vi "lineStartEndInfo.vi"(9 "current location":T1, 10 "line status":cluster{"line start":bool, "line end":bool}, 11 "scan info":T2) -> (3 "scan info out":T2)   [LabVIEW 2010]
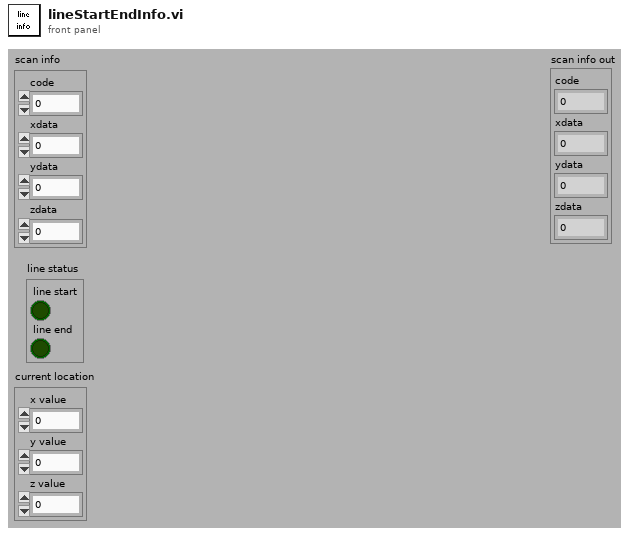
[diagram p1: front panel]
types:
  T1 = cluster{"x value":i16, "y value":i16, "z value":i16}
  T2 = cluster{"code":i32, "xdata":i32, "ydata":i32, "zdata":i32}
  T3 = enum16{"NONE", "VOLUME_START", "LINE_START", "LINE_END", "VOLUME_END"}
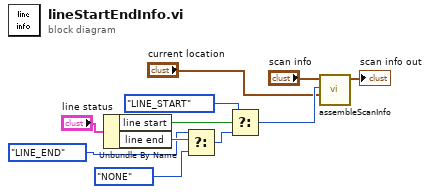
[diagram p0: block diagram]
diagram:
  n1 = Unbundle By Name("line status") -> ("line start"=w8:bool, "line end"=w7:bool)
  n2 = Select(t=T3."LINE_END", s=w7, f=T3."NONE" ("message")) -> (s? t:f=w6:T3)
  n3 = Select(t=T3."LINE_START", s=w8, f=w6) -> (s? t:f=w2:T3)
  n4 = call "assembleScanInfo.vi"("current location/com/max vals"="current location", "message"=w2, "scan info"="scan info") -> ("scan info out"=→"scan info out":T2)  [unwired: 8 in]
